vi "Build Major Frame End.vi"(7 "Virtual Memory Unit in":refnum<class "Virtual Memory Unit.lvclass">, 8 "error in (no error)":errorcluster, 10 "Starting Address":u16 format="%04x", 11 "Major Frame in":refnum<class "Major Frame.lvclass">) -> (0 "error out":errorcluster, 2 "Next Available Address":u16 format="%04x", 3 "Major Frame out":refnum<class "Major Frame.lvclass">, 5 "Virtual Memory Unit out":refnum<class "Virtual Memory Unit.lvclass">)   [LabVIEW 2020, in "BCI-1553 API.lvlib" / "Major Frame.lvclass"]
doc: "The last few commands of the Major Frame will be to wait out the minor frame timer and return to the start of the Major Frame schedule."
uses:
  Major Frame.lvclass
  Dependencies/Virtual Memory Unit/Virtual Memory Unit.lvclass
  TypeDefs/BC Op Codes - Verbose.ctl
  TypeDefs/BC Condition Codes.ctl
  Major Frame.lvclass/Major Frame.ctl
  BCI-1553 API.lvlib
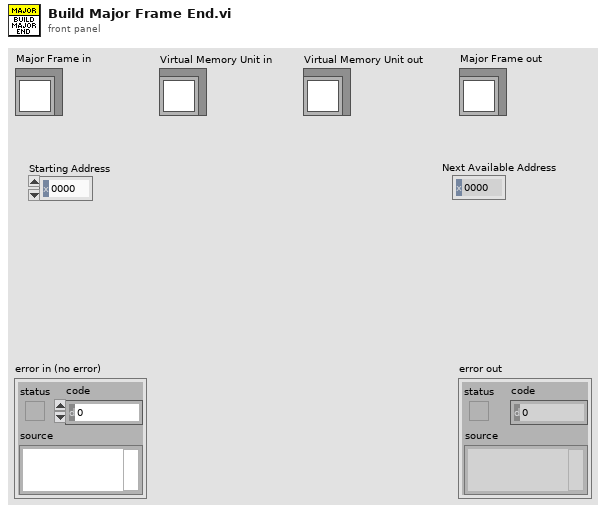
[diagram p1: front panel]
types:
  T1 = typedef "BCI-1553 API.lvlib/BC Condition Codes.ctl" = enum16{"GP0 == 1 || LT", "GP1 == 1 || NE", "GP2 == 1", "GP3 == 1", "GP4 == 1", "GP5 == 1", "GP6 == 1", "GP7 == 1", "NORESP", "FMTERR", "GOODBLOCK", "MSKSTATSET", "BADMSG", "1RETRY", "2RETRY", "ALWAYS"}
  T2 = typedef "BCI-1553 API.lvlib/BC Op Codes - Verbose.ctl" = enum16{"EXECUTE MSG", "EXECUTE MSG GO", "JUMP", "CALL SUBROUTINE", "RETURN", "INTERRUPT REQUEST", "HALT", "DELAY", "WAIT FRAME TIMER = 0", "COMPARE FRAME TIMER", "COMPARE MSG TIMER", "LOAD TIME TAG CTR", "LOAD TIME TAG CTR HI", "LOAD FRAME TIMER", "START FRAME TIMER", "PUSH TIME TAG COUNT", "PUSH TIME TAG COUNT HI", "PUSH TIME TAG COUNT BOTH", "PUSH BLOCK STATUS WORD", "PUSH CURRENT VALUE", "PUSH INDIRECT", "WAIT EXT TRIGGER", "EXECUTE AND FLIP", "EXECUTE, FLIP, GO", "WRITE VALUE TO WMI", "WRITE VALUE TO MEM", "DECREMENT RAM, SKIP", "FLAG"}
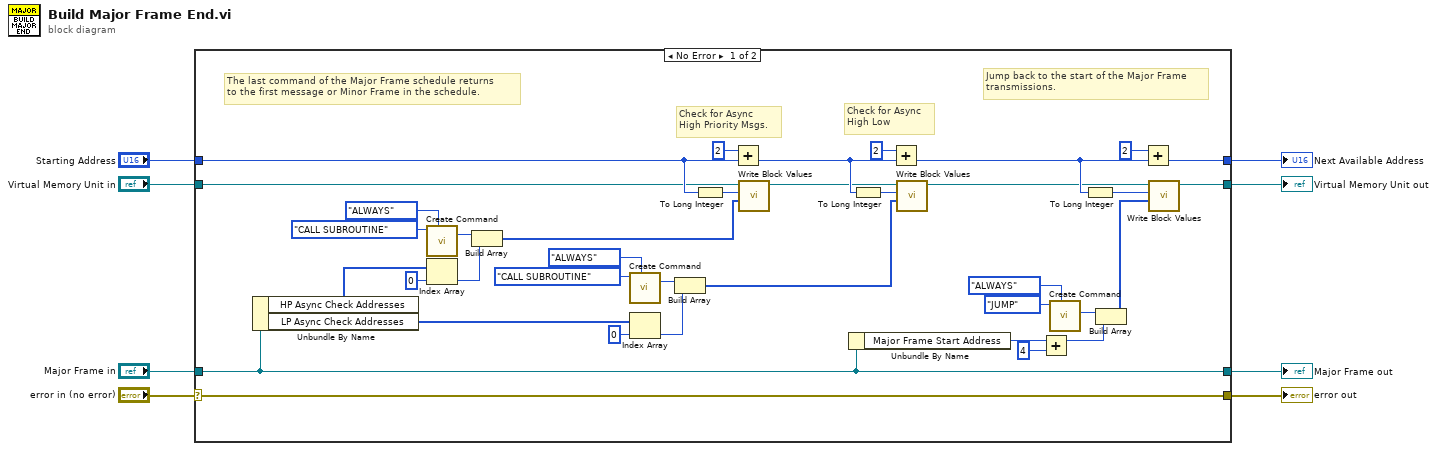
[diagram p0: block diagram]
diagram:
  n1 = case shown="No Error" "error in (no error)" {
    selector: "error in (no error)" -> [w45 w49]
    tunnel: [w45 w49] -> w1
    tunnel: [w33 w48] -> w2
    tunnel: "Major Frame in" -> [w33 w48]
    tunnel: [w37 w46] -> w3
    tunnel: "Virtual Memory Unit in" -> [w22 w46]
    tunnel: [w38 w47] -> w4
    tunnel: "Starting Address" -> [w26 w47]
    frame No Error {
      # "Check for Async\nHigh Low"
      # "Check for Async\nHigh Priority Msgs."
      # "Jump back to the start of the Major Frame\ntransmissions."
      # "The last command of the Major Frame schedule returns\nto the first message or Minor Frame in the schedule."
      n2 = Unbundle By Name(w33) -> ("HP Async Check Addresses"=w25:u16[], "LP Async Check Addresses"=w16:u16[])
      n3 = call "Create Command.vi"("Condition"=BC_Condition_Codes."ALWAYS", "Op Code"=BC_Op_Codes_-_Verbose."CALL SUBROUTINE") -> ("Instruction"=w31:u16)  [unwired: 8 in, 1 out]
      n4 = Index Array(array=w25, index=0) -> (element=w24:u16)
      n5 = Build Array(w31, w24) -> (w32:u16[])
      n6 = call "Create Command.vi"("Condition"=BC_Condition_Codes."ALWAYS", "Op Code"=BC_Op_Codes_-_Verbose."CALL SUBROUTINE") -> ("Instruction"=w17:u16)  [unwired: 8 in, 1 out]
      n7 = Index Array(array=w16, index=0) -> (element=w20:u16)
      n8 = Build Array(w17, w20) -> (w12:u16[])
      n9 = To Long Integer(number=w26) -> (32bit integer=w28:i32)
      n10 = Add(x=u16 2, y=w26) -> (x+y=w11:u16)
      n11 = call "Write Block Values.vi"("Write Block"=w32, "Start Index"=w28, "Virtual Memory Unit in"=w22) -> ("Virtual Memory Unit out"=w10:refnum<class "Virtual Memory Unit.lvclass">)  [unwired: 7 in, 1 out]
      n12 = Unbundle By Name(w33) -> ("Major Frame Start Address"=w36:u16)
      n13 = To Long Integer(number=w11) -> (32bit integer=w14:i32)
      n14 = Add(x=u16 2, y=w11) -> (x+y=w13:u16)
      n15 = call "Write Block Values.vi"("Write Block"=w12, "Start Index"=w14, "Virtual Memory Unit in"=w10) -> ("Virtual Memory Unit out"=w9:refnum<class "Virtual Memory Unit.lvclass">)  [unwired: 7 in, 1 out]
      n16 = Add(x=w36, y=u16 4) -> (x+y=w35:u16)
      n17 = call "Create Command.vi"("Condition"=BC_Condition_Codes."ALWAYS", "Op Code"=BC_Op_Codes_-_Verbose."JUMP") -> ("Instruction"=w41:u16)  [unwired: 8 in, 1 out]
      n18 = To Long Integer(number=w13) -> (32bit integer=w43:i32)
      n19 = Build Array(w41, w35) -> (w44:u16[])
      n20 = Add(x=u16 2, y=w13) -> (x+y=w38:u16)
      n21 = call "Write Block Values.vi"("Write Block"=w44, "Start Index"=w43, "Virtual Memory Unit in"=w9) -> ("Virtual Memory Unit out"=w37:refnum<class "Virtual Memory Unit.lvclass">)  [unwired: 7 in, 1 out]
    }
    frame Error {
    }
  }
  "error out" <- w1
  "Major Frame out" <- w2
  "Virtual Memory Unit out" <- w3
  "Next Available Address" <- w4
